vi "(SubVI) Get Real Position _PI_YCC.vi"(4 "Axis":i32) -> (1 "Real Current Commanded position (um)":dbl format="%0.5f")   [LabVIEW 2014]
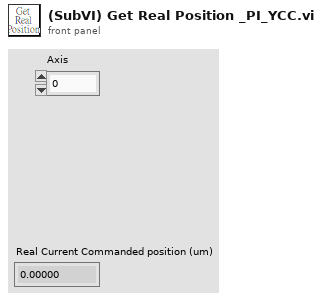
[diagram p1: front panel]
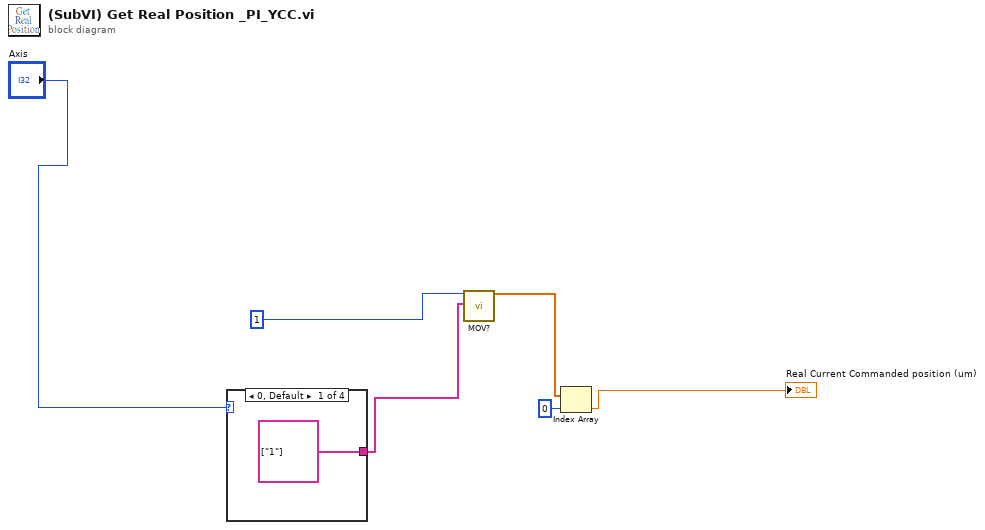
[diagram p0: block diagram]
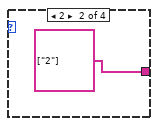
[diagram p2: hidden frame]
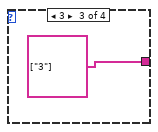
[diagram p3: hidden frame]
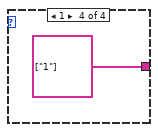
[diagram p4: hidden frame]
diagram:
  n1 = case shown="0, Default" "Axis" {
    tunnel: [string[] ["1"] string[] ["2"] string[] ["3"] string[] ["1"]] -> w3
    frame 0, Default {
    }
    frame 2 {
    }
    frame 3 {
    }
    frame 1 {
    }
  }
  n2 = call "MOV?.vi"("System no."=1, "Axes to query"=w3) -> ("Target position"=w2:dbl[])  [unwired: 16 in, 1 out]
  n3 = Index Array(array=w2, index=0) -> (element=→"Real Current Commanded position (um)":dbl)
